vi "Scale Encoder Counts to Inches.vi"(11 "Target Height (in)":dbl) -> (3 "Encoder Counts":dbl)   [LabVIEW 2017]
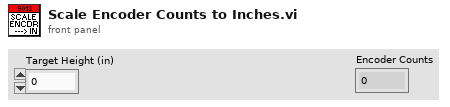
[diagram p1: front panel]
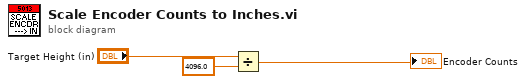
[diagram p0: block diagram]
diagram:
  n1 = Divide(x="Target Height (in)", y=4096.0 ("x")) -> (x/y=→"Encoder Counts":dbl)
